vi "TLB Native Dynamic Events ver 0.06 alpha.vi"() -> ()   [LabVIEW 2018]
uses:
  Labview Training Phase 2/Enum Controls/States for Action Engine.ctl
  Type def/TLB event states.ctl
  Type def/TLB MHL States.ctl
  <vilib>/Studica/Studica Toolkit/NavX/NavX.lvlib
  <vilib>/Studica/Studica Toolkit/Background/I2C Channel.ctl
  <vilib>/myRIO/Common/Instrument Driver Framework/myRIO v1.0/AI/typedefs/AI Channels Enum.ctl
  <vilib>/myRIO/Common/Instrument Driver Framework/myRIO v1.0/AI/typedefs/AI Channels List.ctl
  <vilib>/Studica/Studica Toolkit/Background/Mxp Selection.ctl
  <vilib>/ptbypt/NI_PtbyPt.lvlib
panel:
  out "Waveform Chart 3":dbl(graph)
  out "mean":dbl format="%0.2f"
  out "CM":fxp<+,64,16>
  out "wDistance":dbl
  out "xDistance":dbl
  out "yDistance":dbl
  in  "Reset Encoder 0":bool
  out "Speed":T1
  in  "wTargetSpeed":dbl
  in  "yTargetSpeed":dbl
  in  "xTargetSpeed":dbl
  out "Sharp IR Distance 2":dbl
  out "Sharp IR Distance":dbl
  out "YRPHfH":T2
  out "Displacement":T3
  out "LinearAcceleration":T4
  out "NavX Info Out":T6
  out "Action Queues":string[](array[string])
  out "State logic":T7
  out "Action State":string
  in  "Task condition":bool
  in  "Combo Box":string(combo)
  in  "Stop Queue":bool
  in  "Start Task":bool
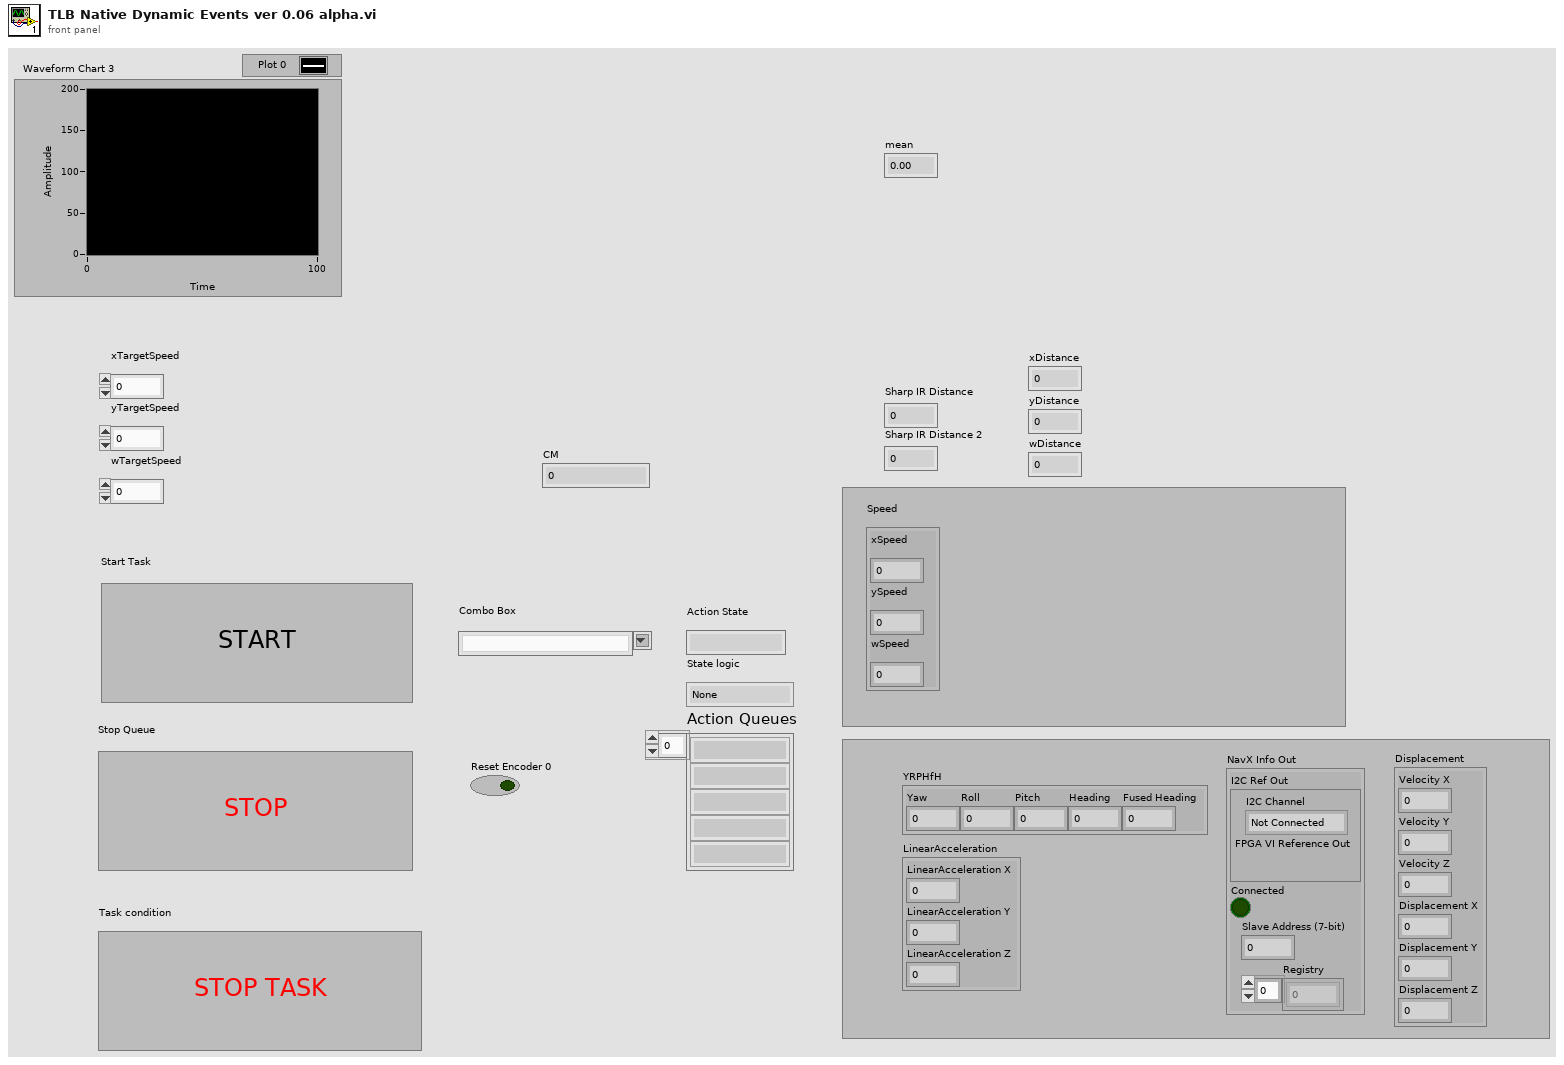
[diagram p1: front panel]
types:
  T1 = cluster{"xSpeed":dbl, "ySpeed":dbl, "wSpeed":dbl}
  T2 = cluster{"Yaw":dbl, "Roll":dbl, "Pitch":dbl, "Heading":dbl, "Fused Heading":dbl}
  T3 = cluster{"Velocity X":dbl, "Velocity Y":dbl, "Velocity Z":dbl, "Displacement X":dbl, "Displacement Y":dbl, "Displacement Z":dbl}
  T4 = cluster{"LinearAcceleration X":dbl, "LinearAcceleration Y":dbl, "LinearAcceleration Z":dbl}
  T5 = typedef "I2C Channel.ctl" = enum16{"Not Connected", "A", "B"}
  T6 = cluster{"I2C Ref Out":cluster{"I2C Channel":T5, "FPGA VI Reference Out":refnum<k20>}, "Connected":bool, "Slave Address (7-bit)":u8, "Registry":u8[]}
  T7 = typedef "TLB MHL States.ctl" = enum16{"None", "Startup", "Idle", "Processing", "Shutdown", "Reset", "Task 1", "Task 2", "Task 3", "Task 4", "Task 4a", "Task 4b", "Task 4c", "Task 4d", "Task 4e", "Task 4f", "Task 4g", "Task 4h", "Acquire image", "Wall follow mode", "Drive Straight"}
  T8 = typedef "States for Action Engine.ctl" = enum16{"Initialize", "Write", "Read"}
  T9 = typedef "TLB event states.ctl" = enum16{"Start Sequence", "Exit", "Start Task 1", "Start Task 2", "Start Task 3", "Start Task 4", "Camera vision", "Wall follow mode", "Idle", "Start Drive Straight"}
  T10 = typedef "Mxp Selection.ctl" = enum16{"MXP A", "MXP B"}
  T11 = typedef "TLB event states.ctl" = enum16{"Start Sequence", "Exit", "Task 1", "Task 2", "Idle"}
  T12 = cluster{"queue out":refnum<queue>, "error out":errorcluster}
  T13 = cluster{"xDistance":dbl, "yDistance":dbl, "wDistance":dbl}
  T14 = typedef "AI Channels List.ctl" = T15[]
  T15 = typedef "AI Channels Enum.ctl" = enum16{"Not Connected", "AudioIn/Left", "AudioIn/Right", "C/AI0", "C/AI1", "A/AI0", "A/AI1", "A/AI2", "A/AI3", "A/AI4", "A/AI5", "A/AI6", "A/AI7", "B/AI0", "B/AI1", "B/AI2", "B/AI3", "B/AI4", "B/AI5", "B/AI6", "B/AI7", "AI/AI0", "AI/AI1", "AI/AI2", "AI/AI3", "A/AI0 (DIFF)", "A/AI1 (DIFF)", "A/AI2 (DIFF)", "A/AI3 (DIFF)", "B/AI0 (DIFF)", "B/AI1 (DIFF)", "B/AI2 (DIFF)", "B/AI3 (DIFF)"}
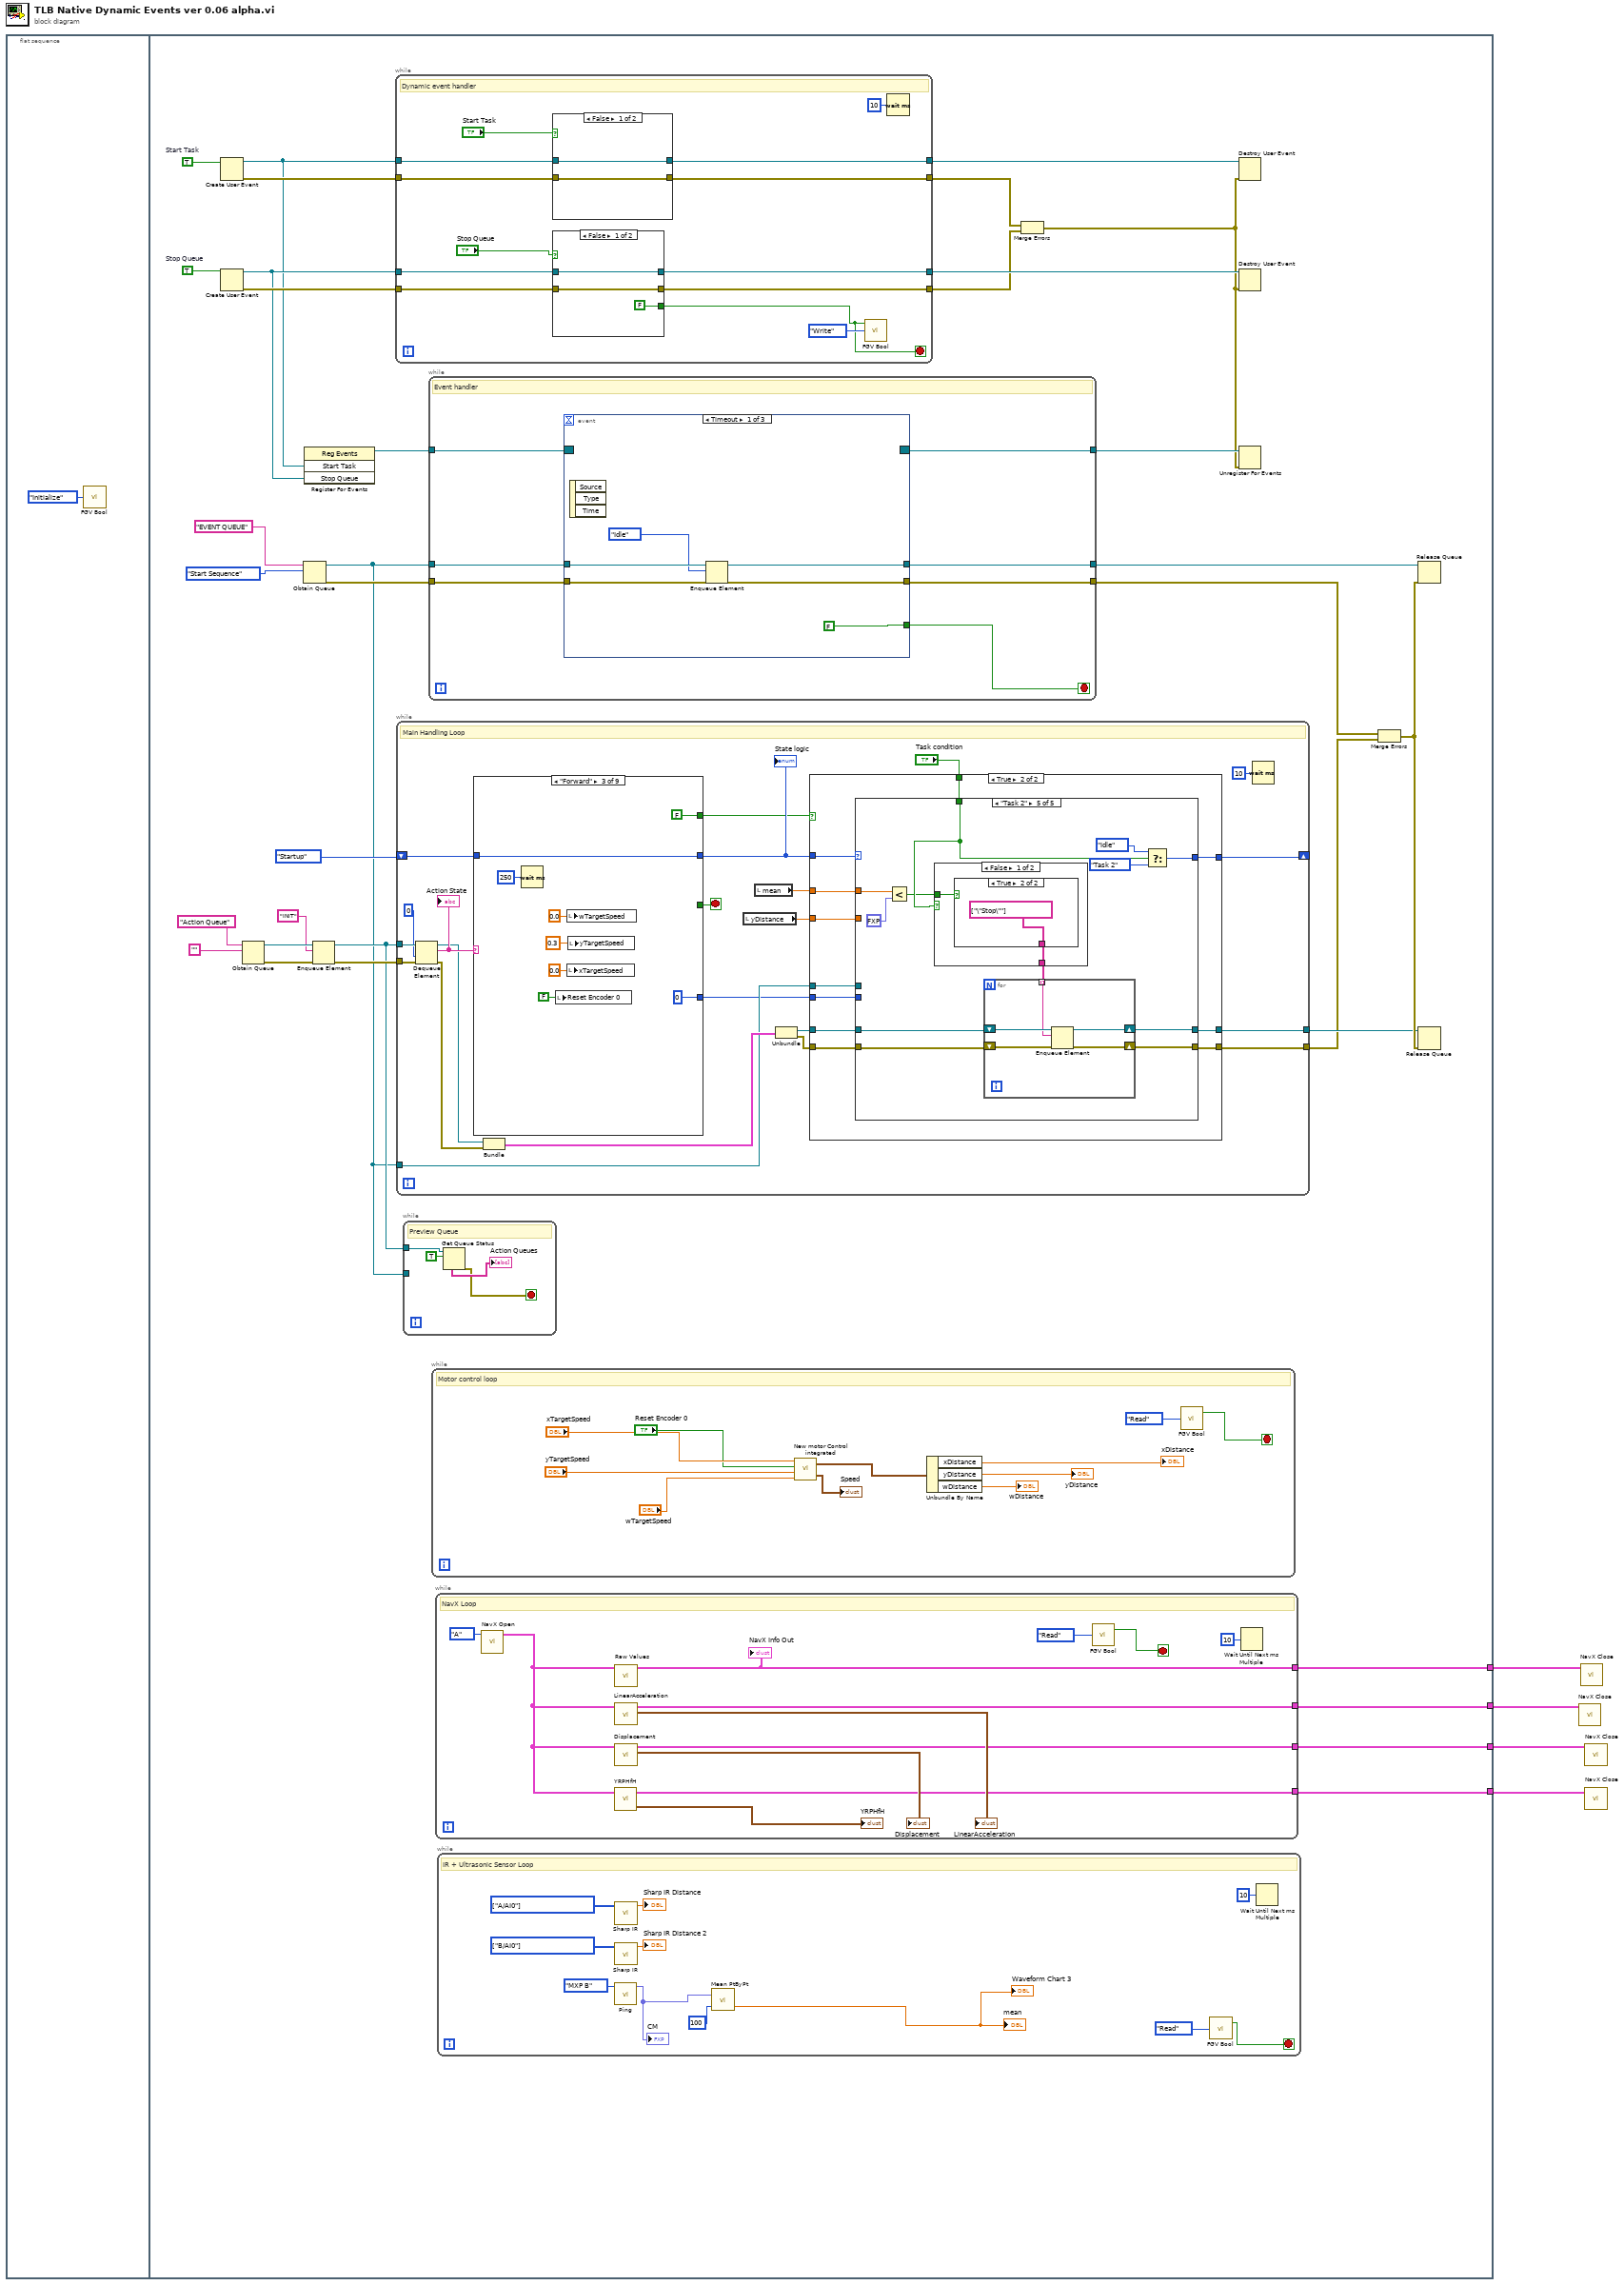
[diagram p0: block diagram]
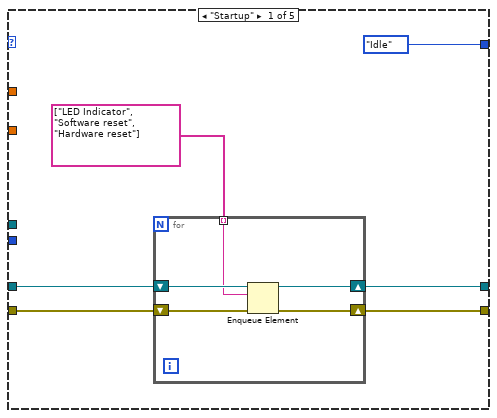
[diagram p3: hidden frame]
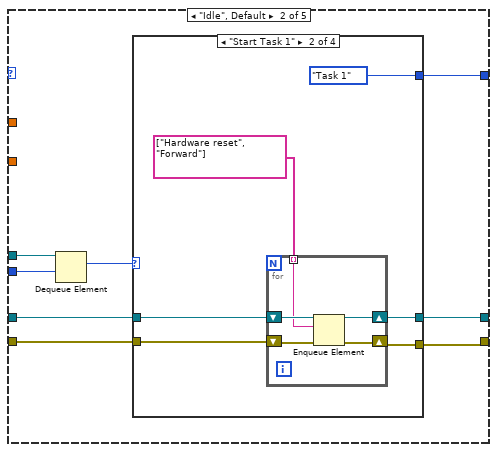
[diagram p4: hidden frame]
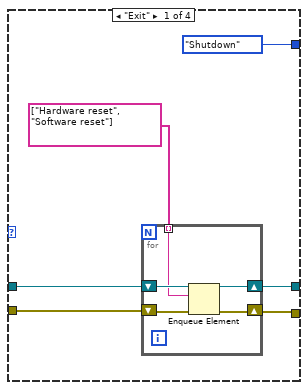
[diagram p5: hidden frame]
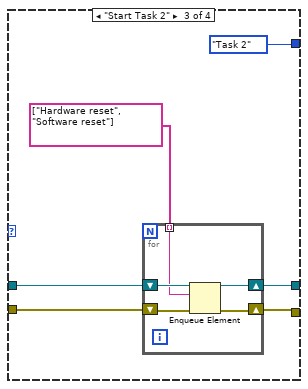
[diagram p6: hidden frame]
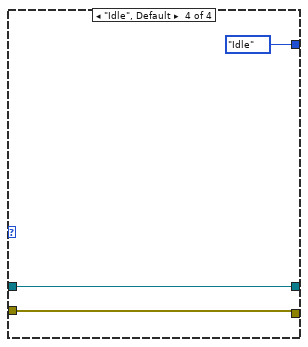
[diagram p7: hidden frame]
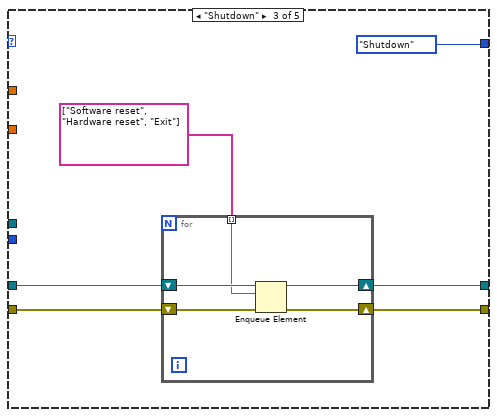
[diagram p8: hidden frame]
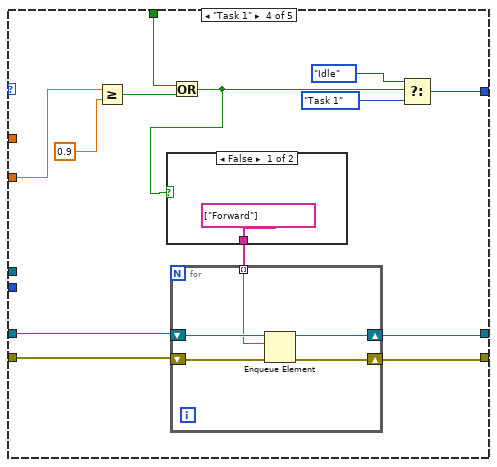
[diagram p9: hidden frame]
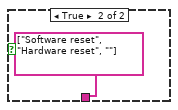
[diagram p10: hidden frame]
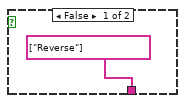
[diagram p11: hidden frame]
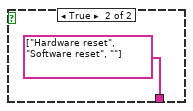
[diagram p12: hidden frame]
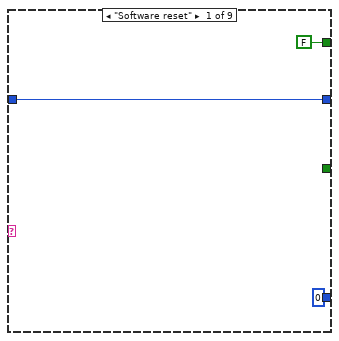
[diagram p13: hidden frame]
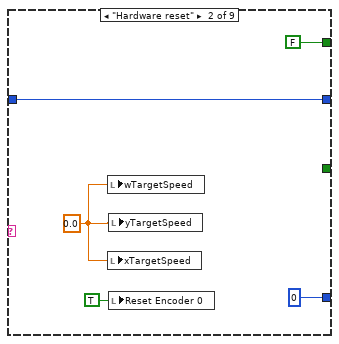
[diagram p14: hidden frame]
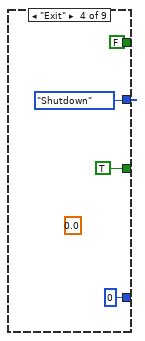
[diagram p15: hidden frame]
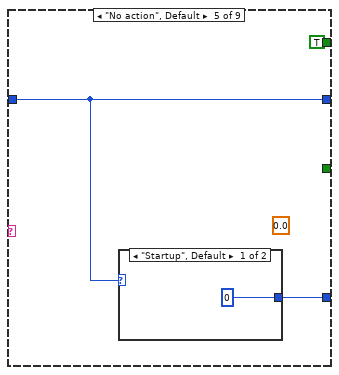
[diagram p16: hidden frame]
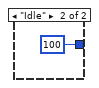
[diagram p17: hidden frame]
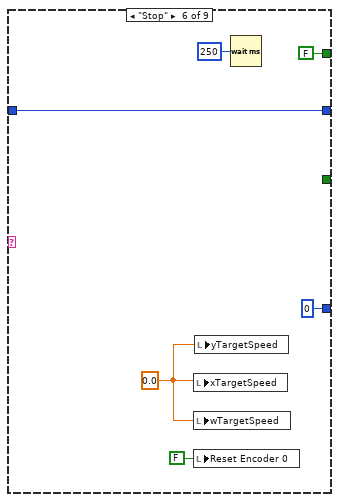
[diagram p18: hidden frame]
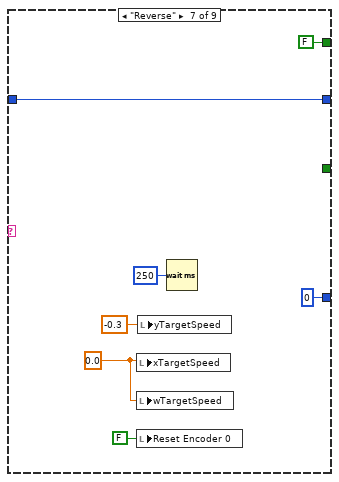
[diagram p19: hidden frame]
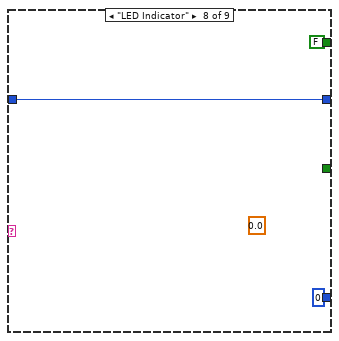
[diagram p20: hidden frame]
diagram:
  n1 = flat-sequence {
    tunnel: [w9] -> w4
    tunnel: [w8] -> w3
    tunnel: [w7] -> w2
    tunnel: [w6] -> w1
    frame #0 {
      n2 = call "FGV Bool.vi"("Init/Read/Write State"=States_for_Action_Engine."Initialize") -> ()  [unwired: 2 in, 2 out]
    }
    frame #1 {
      w39 = TRUE  # Stop Queue
      w38 = TRUE  # Start Task
      n3 = Create User Event(user event datatype=w38) -> (user event=w30:refnum<user-event>, error out=w35:errorcluster)  [unwired: 1 in]
      n4 = Create User Event(user event datatype=w39) -> (user event=w31:refnum<user-event>, error out=w34:errorcluster)  [unwired: 1 in]
      n5 = Obtain Queue(name (unnamed)="Action Queue", element data type="") -> (queue out=w23:refnum<queue>, error out=w19:errorcluster)  [unwired: 3 in, 1 out]
      n6 = Obtain Queue(name (unnamed)="EVENT QUEUE", element data type=TLB_event_states."Start Sequence" ("Enum")) -> (queue out=w10:refnum<queue>, error out=w20:errorcluster)  [unwired: 3 in, 1 out]
      n7 = register-events(w30, w31) -> (reference out=w29:refnum<event-registration>)  [unwired: 2 in, 1 out]
      n8 = Enqueue Element(queue=w23, element="INIT", error in (no error)=w19) -> (queue out=w11:refnum<queue>, error out=w18:errorcluster)  [unwired: 1 in, 1 out]
      n9 = while {
        tunnel: w30 -> [w305]
        tunnel: w31 -> [w304]
        tunnel: [w303] -> w37
        tunnel: [w302] -> w36
        tunnel: w35 -> [w301]
        tunnel: [w300] -> w33
        tunnel: w34 -> [w299]
        tunnel: [w298] -> w32
        stop <- w294 stop-if-true
        # "Dynamic event handler"
        n10 = case shown="False" "Start Task" {
          selector: "Start Task" -> [_ w317]
          tunnel: w305 -> [w316 w321]
          tunnel: [w316 w320] -> w302
          tunnel: w301 -> [w315 w319]
          tunnel: [w315 w318] -> w300
          frame False {
          }
          frame True {
            n11 = Generate User Event(user event=w321, event data cluster=w317, error in=w319) -> (user event out=w320:refnum<user-event>, error out=w318:errorcluster)  [unwired: 1 in]
          }
        }
        n12 = case shown="False" "Stop Queue" {
          selector: "Stop Queue" -> [_ w310]
          tunnel: w304 -> [w309 w314]
          tunnel: [w309 w313] -> w303
          tunnel: w299 -> [w308 w312]
          tunnel: [w308 w311] -> w298
          tunnel: [FALSE w310] -> w294
          frame False {
          }
          frame True {
            n13 = Generate User Event(user event=w314, event data cluster=w310, error in=w312) -> (user event out=w313:refnum<user-event>, error out=w311:errorcluster)  [unwired: 1 in]
          }
        }
        n14 = call "FGV Bool.vi"("Init/Read/Write State"=States_for_Action_Engine."Write", "Input Node"=w294) -> ()  [unwired: 1 in, 2 out]
        n15 = Wait (ms)(milliseconds to wait=u32 10) -> ()  [unwired: 1 out]
      }
      n16 = while {
        tunnel: w10 -> [w85]
        shift-right: [w86] -> _
        shift-left: TLB_MHL_States."Startup" ("Enum") -> [w98]
        tunnel: w11 -> [w96]
        tunnel: w18 -> [w94]
        tunnel: [w88] -> w15
        tunnel: [w87] -> w14
        stop <- w83 stop-if-true
        # "Main Handling Loop"
        n17 = Dequeue Element(queue=w96, timeout in ms (-1)=0, error in (no error)=w94) -> (queue out=w93:refnum<queue>, element=w95:string, error out=w92:errorcluster)  [unwired: 1 out]
        "Action State" <- w95
        n18 = case shown="\"Forward\"" w95 {
          tunnel: [w224 w229 w236 TLB_MHL_States."Shutdown" ("Enum") w244 w252 w258 w262 w265] -> w97
          tunnel: w98 -> [w224 w229 w236 _ w244 w252 w258 w262 w265]
          tunnel: [0 0 0 0 w243 0 0 0 0] -> w84
          tunnel: [_ _ _ TRUE _ _ _ _ _] -> w83
          tunnel: [FALSE FALSE FALSE FALSE TRUE FALSE FALSE FALSE FALSE] -> w81
          frame "Software reset" {
          }
          frame "Hardware reset" {
            w226 = 0.0
            n19 = local write "wTargetSpeed"(w226) -> ()
            n20 = local write "xTargetSpeed"(w226) -> ()
            n21 = local write "yTargetSpeed"(w226) -> ()
            n22 = local write "Reset Encoder 0"(TRUE ("Reset Encoder 0")) -> ()
          }
          frame "Forward" {
            n23 = Wait (ms)(milliseconds to wait=u32 250) -> ()  [unwired: 1 out]
            n24 = local write "Reset Encoder 0"(FALSE ("Reset Encoder 0")) -> ()
            n25 = local write "wTargetSpeed"(0.0 ("wTargetSpeed")) -> ()
            n26 = local write "xTargetSpeed"(0.0 ("xTargetSpeed")) -> ()
            n27 = local write "yTargetSpeed"(0.3 ("yTargetSpeed")) -> ()
          }
          frame "Exit" {
            (unwired) 0.0
          }
          frame "No action", Default {
            (unwired) 0.0
            n28 = case shown="\"Startup\", Default" w244 {
              tunnel: [0 100] -> w243
              frame "Startup", Default {
              }
              frame "Idle" {
              }
            }
          }
          frame "Stop" {
            w249 = 0.0
            n29 = local write "xTargetSpeed"(w249) -> ()
            n30 = local write "wTargetSpeed"(w249) -> ()
            n31 = local write "Reset Encoder 0"(FALSE ("Reset Encoder 0")) -> ()
            n32 = local write "yTargetSpeed"(w249) -> ()
            n33 = Wait (ms)(milliseconds to wait=u32 250) -> ()  [unwired: 1 out]
          }
          frame "Reverse" {
            w255 = 0.0
            n34 = local write "xTargetSpeed"(w255) -> ()
            n35 = local write "wTargetSpeed"(w255) -> ()
            n36 = local write "Reset Encoder 0"(FALSE ("Reset Encoder 0")) -> ()
            n37 = local write "yTargetSpeed"(-0.3 ("yTargetSpeed")) -> ()
            n38 = Wait (ms)(milliseconds to wait=u32 250) -> ()  [unwired: 1 out]
          }
          frame "LED Indicator" {
            (unwired) 0.0
          }
          frame "INIT" {
            (unwired) 0.0
          }
        }
        "State logic" <- w97
        n39 = Bundle("queue out"=w93, "error out"=w92) -> (w91:T12)  [unwired: 1 in]
        n40 = local read "yDistance"() -> (w79:dbl)
        n41 = local read "mean"() -> (w78:dbl)
        n42 = Unbundle(w91) -> ("queue out"=w90:refnum<queue>, "error out"=w89:errorcluster)
        n43 = case shown="True" w81 {
          tunnel: w97 -> [w101 w113]
          tunnel: w90 -> [w102 w112]
          tunnel: w89 -> [w100 w111]
          tunnel: [w102 w110] -> w88
          tunnel: [w100 w109] -> w87
          tunnel: [w101 w108] -> w86
          tunnel: w85 -> [_ w107]
          tunnel: w84 -> [_ w106]
          tunnel: "Task condition" -> [_ w105]
          tunnel: w79 -> [_ w104]
          tunnel: w78 -> [_ w103]
          frame False {
          }
          frame True {
            n44 = case shown="\"Task 2\"" w113 {
              tunnel: w112 -> [w119 w126 w172 w187 w206]
              tunnel: w111 -> [w118 w128 w170 w186 w205]
              tunnel: [w117 w129 w171 w189 w208] -> w110
              tunnel: [w116 w127 w169 w188 w207] -> w109
              tunnel: [TLB_MHL_States."Idle" ("Enum") w130 TLB_MHL_States."Shutdown" ("Enum") w190 w209] -> w108
              tunnel: w107 -> [_ w132 _ _ _]
              tunnel: w106 -> [_ w125 _ _ _]
              tunnel: w105 -> [_ _ _ w184 w204]
              tunnel: w104 -> [_ _ _ w181 _]
              tunnel: w103 -> [_ _ _ _ w202]
              frame "Startup" {
                n45 = for {
                  shift-right: [w122] -> w117
                  shift-left: w119 -> [w124]
                  shift-right: [w121] -> w116
                  shift-left: w118 -> [w123]
                  tunnel: string[] ["LED Indicator", "Software reset", "Hardware reset"] -> [w120] mode=indexing
                  n46 = Enqueue Element(queue=w124, element=w120, error in (no error)=w123) -> (queue out=w122:refnum<queue>, error out=w121:errorcluster)  [unwired: 1 in, 1 out]
                }
              }
              frame "Idle", Default {
                n47 = Dequeue Element(queue=w132, timeout in ms (-1)=w125) -> (element=w131:T9)  [unwired: 1 in, 3 out]
                n48 = case shown="\"Start Task 1\"" w131 {
                  tunnel: [TLB_MHL_States."Shutdown" ("Enum") TLB_MHL_States."Task 1" ("Enum") TLB_MHL_States."Task 2" ("Enum") TLB_MHL_States."Idle" ("Enum")] -> w130
                  tunnel: [w135 w148 w157 w167] -> w129
                  tunnel: w126 -> [w137 w147 w159 w167]
                  tunnel: w128 -> [w136 w146 w158 w166]
                  tunnel: [w134 w145 w156 w166] -> w127
                  frame "Exit" {
                    n49 = for {
                      shift-right: [w143] -> w135
                      shift-left: w137 -> [w142]
                      shift-right: [w140] -> w134
                      shift-left: w136 -> [w141]
                      tunnel: string[] ["Hardware reset", "Software reset"] -> [w139] mode=indexing
                      n50 = Enqueue Element(queue=w142, element=w139, error in (no error)=w141) -> (queue out=w143:refnum<queue>, error out=w140:errorcluster)  [unwired: 1 in, 1 out]
                    }
                  }
                  frame "Start Task 1" {
                    n51 = for {
                      shift-right: [w154] -> w148
                      shift-left: w147 -> [w153]
                      shift-right: [w151] -> w145
                      shift-left: w146 -> [w152]
                      tunnel: string[] ["Hardware reset", "Forward"] -> [w150] mode=indexing
                      n52 = Enqueue Element(queue=w153, element=w150, error in (no error)=w152) -> (queue out=w154:refnum<queue>, error out=w151:errorcluster)  [unwired: 1 in, 1 out]
                    }
                  }
                  frame "Start Task 2" {
                    n53 = for {
                      shift-right: [w165] -> w157
                      shift-left: w159 -> [w164]
                      shift-right: [w162] -> w156
                      shift-left: w158 -> [w163]
                      tunnel: string[] ["Hardware reset", "Software reset"] -> [w161] mode=indexing
                      n54 = Enqueue Element(queue=w164, element=w161, error in (no error)=w163) -> (queue out=w165:refnum<queue>, error out=w162:errorcluster)  [unwired: 1 in, 1 out]
                    }
                  }
                  frame "Idle", Default {
                  }
                }
              }
              frame "Shutdown" {
                n55 = for {
                  shift-right: [w177] -> w171
                  shift-left: w172 -> [w179]
                  shift-right: [w176] -> w169
                  shift-left: w170 -> [w178]
                  tunnel: string[] ["Software reset", "Hardware reset", "Exit"] -> [w175] mode=indexing
                  n56 = Enqueue Element(queue=w179, element=w175, error in (no error)=w178) -> (queue out=w177:refnum<queue>, error out=w176:errorcluster)  [unwired: 1 in, 1 out]
                }
              }
              frame "Task 1" {
                n57 = Greater Or Equal?(x=w181, y=0.9 ("x")) -> (x >= y?=w183:bool)
                n58 = Or(x=w184, y=w183) -> (x .or. y?=w182:bool)
                n59 = case shown="False" w182 {
                  tunnel: [string[] ["Forward"] string[] ["Software reset", "Hardware reset", ""]] -> w185
                  frame False {
                  }
                  frame True {
                  }
                }
                n60 = for {
                  shift-right: [w197] -> w189
                  shift-left: w187 -> [w199]
                  shift-right: [w196] -> w188
                  shift-left: w186 -> [w198]
                  tunnel: w185 -> [w195] mode=indexing
                  n61 = Enqueue Element(queue=w199, element=w195, error in (no error)=w198) -> (queue out=w197:refnum<queue>, error out=w196:errorcluster)  [unwired: 1 in, 1 out]
                }
                n62 = Select(t=TLB_MHL_States."Idle" ("Enum"), s=w182, f=TLB_MHL_States."Task 1" ("Enum")) -> (s? t:f=w190:T7)
              }
              frame "Task 2" {
                n63 = Less?(x=w202, y=fxp<+,64,16> 20.0) -> (x < y?=w200:bool)
                n64 = case shown="False" w204 {
                  tunnel: [w212 string[] ["Hardware reset", "Software reset", ""]] -> w203
                  tunnel: w200 -> [w213 _]
                  frame False {
                    n65 = case shown="True" w213 {
                      tunnel: [string[] ["Reverse"] string[] ["\"Stop\""]] -> w212
                      frame False {
                      }
                      frame True {
                      }
                    }
                  }
                  frame True {
                  }
                }
                n66 = for {
                  shift-right: [w219] -> w208
                  shift-left: w206 -> [w221]
                  shift-right: [w218] -> w207
                  shift-left: w205 -> [w220]
                  tunnel: w203 -> [w217] mode=indexing
                  n67 = Enqueue Element(queue=w221, element=w217, error in (no error)=w220) -> (queue out=w219:refnum<queue>, error out=w218:errorcluster)  [unwired: 1 in, 1 out]
                }
                n68 = Select(t=TLB_MHL_States."Idle" ("Enum"), s=w204, f=TLB_MHL_States."Task 2" ("Enum")) -> (s? t:f=w209:T7)
              }
            }
          }
        }
        n69 = Wait (ms)(milliseconds to wait=u32 10) -> ()  [unwired: 1 out]
      }
      n70 = while {
        tunnel: w11 -> [w75]
        tunnel: w10 -> [_]
        stop <- w74 stop-if-true
        # "Preview Queue"
        n71 = Get Queue Status(queue=w75, return elements? (F)=TRUE) -> (error out=w74:errorcluster, elements=→"Action Queues":string[])  [unwired: 1 in, 6 out]
      }
      n72 = while {
        tunnel: w29 -> [w272]
        tunnel: [w271] -> w28
        tunnel: w10 -> [w269]
        tunnel: [w268] -> w27
        tunnel: w20 -> [w267]
        tunnel: [w266] -> w17
        stop <- w270 stop-if-true
        # "Event handler"
        n73 = event shown="[0] Timeout" {
          selector: w272 -> [_ _ _]
          dyn-events: [_ _ _] -> w271
          timeout: _ -> [_ _ _]
          tunnel: [FALSE FALSE w293] -> w270
          tunnel: w269 -> [w277 w284 w291]
          tunnel: [w276 w283 w292] -> w268
          tunnel: w267 -> [w274 w280 w289]
          tunnel: [w273 w279 w288] -> w266
          event Timeout {
            n74 = event-data() -> ()  [unwired: 1 in, 3 out]
            n75 = Enqueue Element(queue=w277, element=TLB_event_states."Idle" ("Enum"), error in (no error)=w274) -> (queue out=w276:refnum<queue>, error out=w273:errorcluster)  [unwired: 1 in, 1 out]
          }
          event User Event {
            n76 = event-data() -> ()  [unwired: 1 in, 5 out]
            n77 = case shown="\"Task 1\", Default" "Combo Box" {
              tunnel: [TLB_event_states."Task 2" ("Enum") TLB_event_states."Start Task 1" ("Enum")] -> w281
              frame "Task 2" {
              }
              frame "Task 1", Default {
              }
            }
            n78 = Enqueue Element(queue=w284, element=w281, error in (no error)=w280) -> (queue out=w283:refnum<queue>, error out=w279:errorcluster)  [unwired: 1 in, 1 out]
          }
          event User Event {
            n79 = event-data() -> ("Stop Queue"=w293:bool)  [unwired: 1 in, 4 out]
            n80 = Enqueue Element(queue=w291, element=TLB_event_states."Exit" ("Enum"), error in (no error)=w289) -> (queue out=w292:refnum<queue>, error out=w288:errorcluster)  [unwired: 1 in, 1 out]
          }
        }
      }
      n81 = while {
        stop <- w72 stop-if-true
        # "Motor control loop"
        n82 = call "New motor Control integrated.vi"("wTargetSpeed"="wTargetSpeed", "yTargetSpeed"="yTargetSpeed", "xTargetSpeed"="Reset Encoder 0", "Reset Encoders"="xTargetSpeed") -> ("Speed"=→"Speed":T1, "Distance"=w66:T13)
        n83 = Unbundle By Name(w66) -> ("xDistance"=→"xDistance":dbl, "yDistance"=→"yDistance":dbl, "wDistance"=→"wDistance":dbl)
        n84 = call "FGV Bool.vi"("Init/Read/Write State"=States_for_Action_Engine."Read") -> ("Output node"=w72:bool)  [unwired: 2 in, 1 out]
      }
      n85 = while {
        tunnel: [w59] -> w9
        tunnel: [w55] -> w8
        tunnel: [w54] -> w7
        tunnel: [w53] -> w6
        stop <- w61 stop-if-true
        # "NavX Loop"
        n86 = call <vilib>:"NavX Open.vi"("I2C Channel"=I2C_Channel."A") -> ("NavX Info"=w51:T6)  [unwired: 9 in, 1 out]
        n87 = call <vilib>:"YRPHfH.vi"("NavX Info In"=w51) -> ("YRPHfH"=→"YRPHfH":T2, "NavX Info Out"=w54:T6)  [unwired: 3 in]
        n88 = call <vilib>:"Raw Values.vi"("NavX Info In"=w51) -> ("NavX Info Out"=w59:T6)  [unwired: 8 in, 1 out]
        "NavX Info Out" <- w59
        n89 = call <vilib>:"LinearAcceleration.vi"("NavX Info In"=w51) -> ("LinearAcceleration"=→"LinearAcceleration":T4, "NavX Info Out"=w55:T6)  [unwired: 9 in]
        n90 = call <vilib>:"Displacement.vi"("NavX Info In"=w51) -> ("Displacement"=→"Displacement":T3, "NavX Info Out"=w53:T6)  [unwired: 9 in]
        n91 = call "FGV Bool.vi"("Init/Read/Write State"=States_for_Action_Engine."Read") -> ("Output node"=w61:bool)  [unwired: 2 in, 1 out]
        n92 = Wait Until Next ms Multiple(millisecond multiple=u32 10) -> ()  [unwired: 1 out]
      }
      n93 = while {
        stop <- w44 stop-if-true
        w49 = T14 [enum."B/AI0"] items=["Not Connected", "AudioIn/Left", "AudioIn/Right", "C/AI0", "C/AI1", "A/AI0", "A/AI1", "A/AI2", "A/AI3", "A/AI4", "A/AI5", "A/AI6", "A/AI7", "B/AI0", "B/AI1", "B/AI2", "B/AI3", "B/AI4", "B/AI5", "B/AI6", "B/AI7", "AI/AI0", "AI/AI1", "AI/AI2", "AI/AI3", "A/AI0 (DIFF)", "A/AI1 (DIFF)", "A/AI2 (DIFF)", "A/AI3 (DIFF)", "B/AI0 (DIFF)", "B/AI1 (DIFF)", "B/AI2 (DIFF)", "B/AI3 (DIFF)"] ("AI Channel")
        w50 = T14 [enum."A/AI0"] items=["Not Connected", "AudioIn/Left", "AudioIn/Right", "C/AI0", "C/AI1", "A/AI0", "A/AI1", "A/AI2", "A/AI3", "A/AI4", "A/AI5", "A/AI6", "A/AI7", "B/AI0", "B/AI1", "B/AI2", "B/AI3", "B/AI4", "B/AI5", "B/AI6", "B/AI7", "AI/AI0", "AI/AI1", "AI/AI2", "AI/AI3", "A/AI0 (DIFF)", "A/AI1 (DIFF)", "A/AI2 (DIFF)", "A/AI3 (DIFF)", "B/AI0 (DIFF)", "B/AI1 (DIFF)", "B/AI2 (DIFF)", "B/AI3 (DIFF)"] ("AI Channel")
        # "IR + Ultrasonic Sensor Loop"
        n94 = call <vilib>:"Ping.vi"("Mxp Side"=Mxp_Selection."MXP B") -> ("CM"=w40:fxp<+,64,16>)  [unwired: 8 in, 2 out]
        "CM" <- w40
        n95 = call <vilib>:"Sharp IR.vi"("AI Channel"=w50) -> ("Sharp IR Distance"=→"Sharp IR Distance":dbl)  [unwired: 8 in, 2 out]
        n96 = call <vilib>:"Sharp IR.vi"("AI Channel"=w49) -> ("Sharp IR Distance"=→"Sharp IR Distance 2":dbl)  [unwired: 8 in, 2 out]
        n97 = call <vilib>:"Mean PtByPt.vi"("x"=w40, "sample length"=100) -> ("mean"=→"mean" →"Waveform Chart 3":dbl)  [unwired: 2 in, 1 out]
        n98 = call "FGV Bool.vi"("Init/Read/Write State"=States_for_Action_Engine."Read") -> ("Output node"=w44:bool)  [unwired: 2 in, 1 out]
        n99 = Wait Until Next ms Multiple(millisecond multiple=u32 10) -> ()  [unwired: 1 out]
      }
      n100 = Merge Errors(w33, w32) -> (w13:errorcluster)
      n101 = Destroy User Event(user event=w36, error in=w13) -> ()  [unwired: 1 out]
      n102 = Destroy User Event(user event=w37, error in=w13) -> ()  [unwired: 1 out]
      n103 = Unregister For Events(event registration refnum=w28, error in=w13) -> ()  [unwired: 1 out]
      n104 = Merge Errors(w17, w14) -> (w16:errorcluster)
      n105 = Release Queue(queue=w27, error in (no error)=w16) -> ()  [unwired: 1 in, 3 out]
      n106 = Release Queue(queue=w15, error in (no error)=w16) -> ()  [unwired: 1 in, 3 out]
    }
  }
  n107 = call <vilib>:"NavX Close.vi"("NavX Info In"=w3) -> ()  [unwired: 10 in, 1 out]
  n108 = call <vilib>:"NavX Close.vi"("NavX Info In"=w4) -> ()  [unwired: 10 in, 1 out]
  n109 = call <vilib>:"NavX Close.vi"("NavX Info In"=w1) -> ()  [unwired: 10 in, 1 out]
  n110 = call <vilib>:"NavX Close.vi"("NavX Info In"=w2) -> ()  [unwired: 10 in, 1 out]
